vi "File.Strip Path of VariableNames.vi"(10 "VariablePattern":string="\\$", 11 "Path":path) -> (3 "Path Out":path)   [LabVIEW 2019]
panel:
  out "array of paths":string[](array[string])
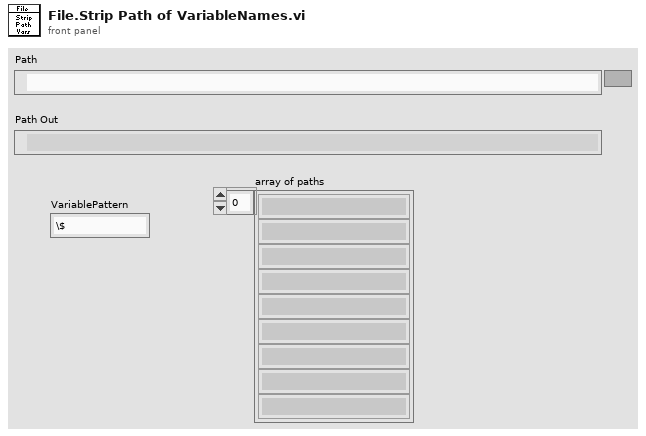
[diagram p1: front panel]
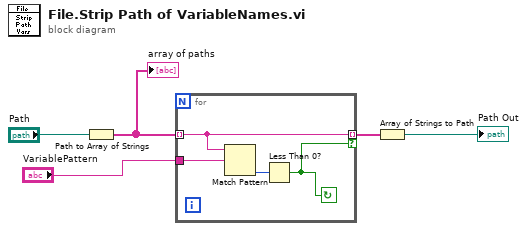
[diagram p0: block diagram]
diagram:
  n1 = Path to Array of Strings(0:"Path") -> (2:w4:string[])  [unwired: 1 out]
  "array of paths" <- w4
  n2 = for {
    tunnel: w4 -> [w9] mode=indexing
    tunnel: [w9] -> w3 mode=indexing if=w7
    tunnel: "VariablePattern" -> [w6]
    stop <- w7 continue-if-true
    n3 = Match Pattern(string=w9, regular expression=w6) -> (offset past match=w8:i32)  [unwired: 1 in, 3 out]
    n4 = Less Than 0?(x=w8) -> (x < 0?=w7:bool)
  }
  n5 = Array of Strings to Path(0:w3) -> (2:→"Path Out":path)  [unwired: 1 in]
